vi "Add Scale.vi"(8 "error in (no error)":errorcluster, 11 "Scaling configuration in":refnum<class "Scaling configuration.lvclass">) -> (0 "error out":errorcluster, 2 "new index":i32, 3 "Scaling configuration out":refnum<class "Scaling configuration.lvclass">)   [LabVIEW 2013, in "Scaling configuration.lvclass"]
uses:
  Scaling configuration.lvclass
  <vilib>/NI/Tag Bus Module Framework/channel/TBM channel.lvclass
  controls/scale data types.ctl
  Scaling configuration.lvclass/Scaling configuration.ctl
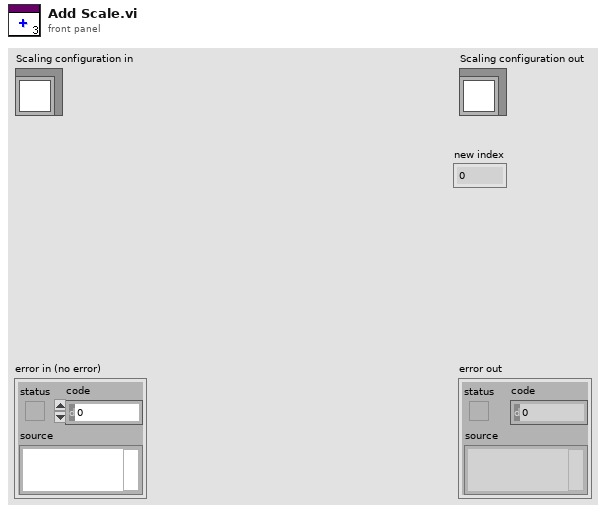
[diagram p1: front panel]
types:
  T1 = typedef "Scaling configuration.lvclass/scale data types.ctl" = enum16{"Double", "Single", "I64", "I32", "I16", "I8", "U64", "U32", "U16", "U8"}
  T2 = cluster{"mappings":cluster{"input channel":refnum<class "TBM channel.lvclass">, "output channel":refnum<class "TBM channel.lvclass">, "input data type":T1, "output data type":T1}[], "name":string}
  T3 = cluster{"mappings":cluster{"input channel":refnum<class "TBM channel.lvclass">, "output channel":refnum<class "TBM channel.lvclass">, "input data type":T1, "output data type":T1}[], "name":string}[]
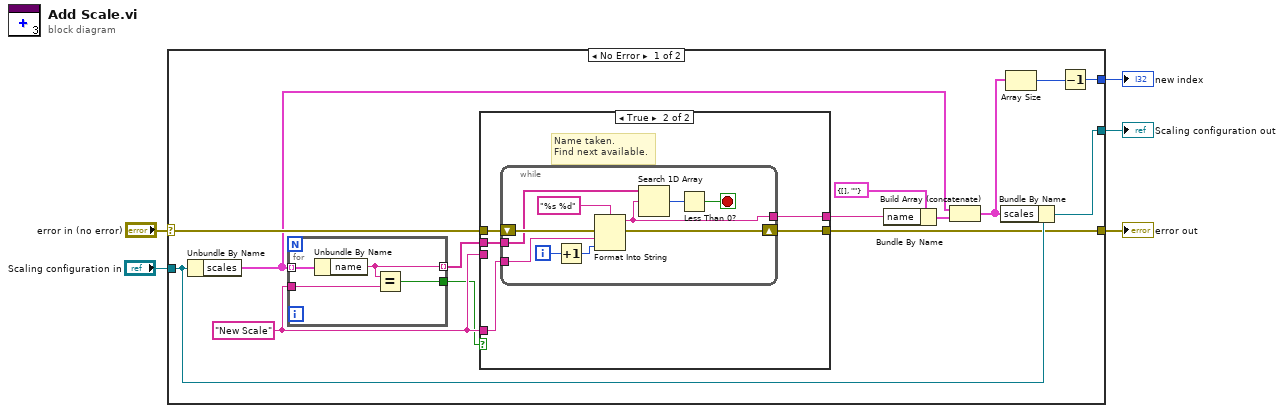
[diagram p0: block diagram]
diagram:
  n1 = case shown="No Error" "error in (no error)" {
    selector: "error in (no error)" -> [w19 w42]
    tunnel: [w16 w42] -> w4
    tunnel: [w17 w41] -> w2
    tunnel: "Scaling configuration in" -> [w18 w41]
    tunnel: [w14 _] -> w1
    frame No Error {
      w13 = "New Scale" ("element")
      n2 = Unbundle By Name(w18) -> ("scales"=w10:T3)
      n3 = for {
        tunnel: w10 -> [w23] mode=indexing
        tunnel: w13 -> [w22]
        tunnel: [w21] -> w12
        tunnel: [w20] -> w11 mode=indexing
        n4 = Unbundle By Name(w23) -> ("name"=w20:string)
        n5 = Equal?(x=w20, y=w22) -> (x = y?=w21:bool)
      }
      n6 = case shown="True" w12 {
        tunnel: [w25 w30] -> w8
        tunnel: [w24 w29] -> w16
        tunnel: w11 -> [_ w28]
        tunnel: w13 -> [_ w27]
        tunnel: w13 -> [w25 _]
        tunnel: w19 -> [w24 w26]
        frame False {
          # "Default name available.\nUse it."
        }
        frame True {
          # "Name taken.\nFind next available."
          n7 = while {
            tunnel: [w35] -> w30
            shift-right: [w33] -> w29
            shift-left: w26 -> [w34]
            tunnel: w28 -> [w32]
            tunnel: w27 -> [w31]
            i -> [w39]
            stop <- w36 stop-if-true
            n8 = Increment(x=w39) -> (x+1=w38:i32)
            n9 = Format Into String(format string="%s %d", error in=w34, w31, w38) -> (resulting string=w35:string, error out=w33:errorcluster)  [unwired: 1 in]
            n10 = Search 1D Array(1D array=w32, element=w35) -> (index of element=w37:i32)  [unwired: 1 in]
            n11 = Less Than 0?(x=w37) -> (x < 0?=w36:bool)
          }
        }
      }
      n12 = Bundle By Name(cluster=T2 {"mappings"=[], "name"=""} ("Cluster"), "name"=w8) -> (w7:T2)
      n13 = Build Array (concatenate)(w10, w7) -> (w6:T3)
      n14 = Bundle By Name(cluster=w18, "scales"=w6) -> (w17:refnum<class "Scaling configuration.lvclass">)
      n15 = Array Size(array=w6) -> (size(s)=w15:i32)
      n16 = Decrement(x=w15) -> (x-1=w14:i32)
    }
    frame Error {
    }
  }
  "error out" <- w4
  "Scaling configuration out" <- w2
  "new index" <- w1
